vi "AssertMultiChannelLoopbackForMappedChannels.vi"(4 "tolerance":dbl=0.01 format="%#_13g", 6 "output values":dbl[](array[numeric]), 7 "delay time (s)":dbl=0.1 format="%#_13g", 8 "error in (no error)":errorcluster, 10 "Map from outputs to inputs":map{string, string[]}(c390), 11 "VeriStand Test Case in":refnum<class "VeriStandTestCase.lvclass">) -> (0 "error out":errorcluster, 3 "VeriStand Test Case out":refnum<class "VeriStandTestCase.lvclass">)   [LabVIEW 2020, in "VeriStandTestCase.lvclass"]
uses:
  VeriStandTestCase.lvclass
  VeriStandTestCase.lvclass/VeriStandTestCase.ctl
  <vilib>/NI VeriStand/Execution/Workspace/NI VeriStand - Get Multiple Channel Values.vi
  <vilib>/NI VeriStand/Execution/Workspace/NI VeriStand - Set Multiple Channel Values.vi
  <vilib>/NI VeriStand/Execution/Workspace/NI_VS Workspace ExecutionAPI.lvlib
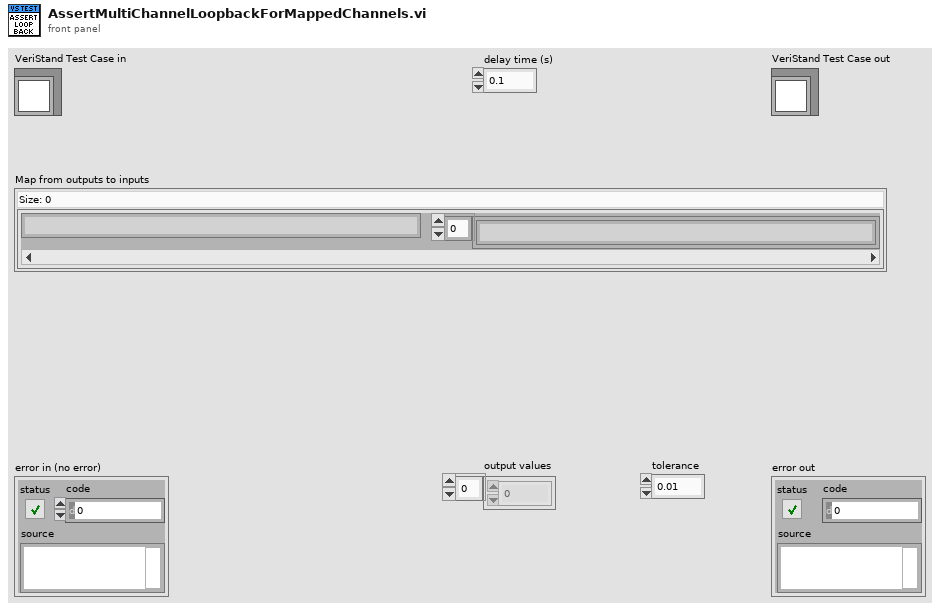
[diagram p1: front panel]
types:
  T1 = typedef "NI_VS Workspace ExecutionAPI.lvlib/WorkspaceAPI.ctl" = refnum<k24>
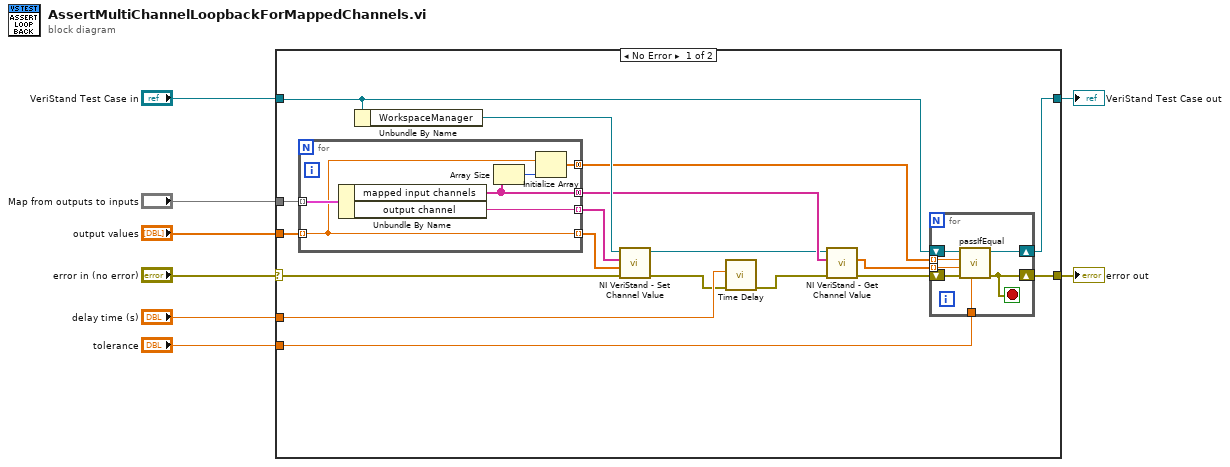
[diagram p0: block diagram]
diagram:
  n1 = case shown="No Error" "error in (no error)" {
    selector: "error in (no error)" -> [w26 w40]
    tunnel: [w10 w40] -> w8
    tunnel: "Map from outputs to inputs" -> [w22 _]
    tunnel: "output values" -> [w19 _]
    tunnel: "delay time (s)" -> [w24 _]
    tunnel: "tolerance" -> [w12 _]
    tunnel: "VeriStand Test Case in" -> [w9 w41]
    tunnel: [w11 w41] -> w3
    frame No Error {
      n2 = for {
        tunnel: w22 -> [w32] mode=indexing
        tunnel: [w28] -> w21 mode=indexing
        tunnel: [w27] -> w20 mode=indexing
        tunnel: w19 -> [w27] mode=indexing
        tunnel: [w30] -> w18 mode=concatenating
        tunnel: [w29] -> w16 mode=concatenating
        n3 = Unbundle By Name(w32) -> ("mapped input channels"=w29:string[], "output channel"=w28:string)
        n4 = Array Size(array=w29) -> (size(s)=w31:i32)
        n5 = Initialize Array(w27, w31) -> (w30:dbl[])
      }
      n6 = Unbundle By Name(w9) -> ("WorkspaceManager"=w23:T1)
      n7 = call-poly <vilib>:"NI VeriStand - Set Channel Value.vi"("error in (no error)"=w26, "Values"=w20, "Channels"=w21, "WorkspaceManager in"=w23) -> ("error out"=w14:errorcluster, "WorkspaceManager out"=w15:T1)  [unwired: 6 in]
      n8 = call "Time Delay"("error in (no error)"=w14, "Delay Time (s)"=w24) -> ("error out"=w25:errorcluster)  [unwired: 9 in]
      n9 = call-poly <vilib>:"NI VeriStand - Get Channel Value.vi"("error in (no error)"=w25, "Channels"=w16, "WorkspaceManager in"=w15) -> ("error out"=w13:errorcluster, "Values"=w17:dbl[])  [unwired: 6 in, 1 out]
      n10 = for {
        tunnel: w12 -> [w38]
        shift-right: [w35] -> w10
        shift-left: w13 -> [w39]
        shift-right: [w37] -> w11
        shift-left: w9 -> [w36]
        tunnel: w18 -> [w34] mode=indexing
        tunnel: w17 -> [w33] mode=indexing
        stop <- w35 stop-if-true
        n11 = call-dynamic "passIfEqual.vi"("delta (optional)"=w38, "error in (no error)"=w39, "y"=w33, "x"=w34, "TestCase in"=w36) -> ("error out"=w35:errorcluster, "TestCase out"=w37:refnum<class "VeriStandTestCase.lvclass">)  [unwired: 5 in]
      }
    }
    frame Error {
    }
  }
  "error out" <- w8
  "VeriStand Test Case out" <- w3
